vi "02_CheckoutBook.vi"() -> ()   [LabVIEW 2020]
uses:
  librarian_class/librarian.lvclass
  client_class/client.lvclass
panel:
  out "Recieved Match?":bool
  in  "book title":string="ProjectGutenberg-64317-TheGreatGatsby.txt"
  out "book contents":string
  in  "timeout in ms (-1)":i32=-1
  out "client error out":errorcluster
  out "lib error out":errorcluster
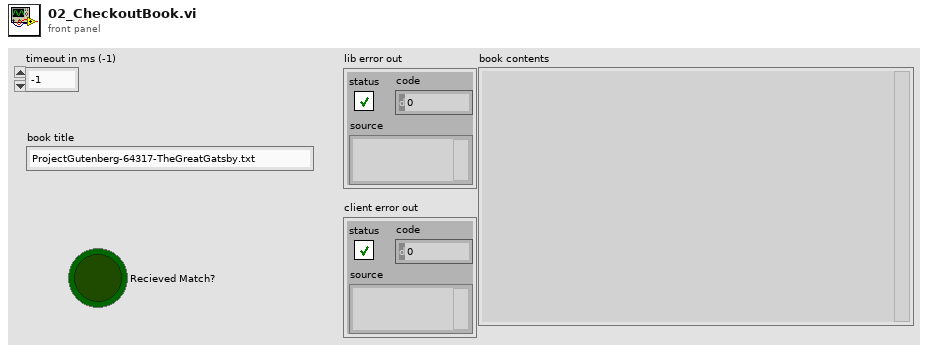
[diagram p1: front panel]
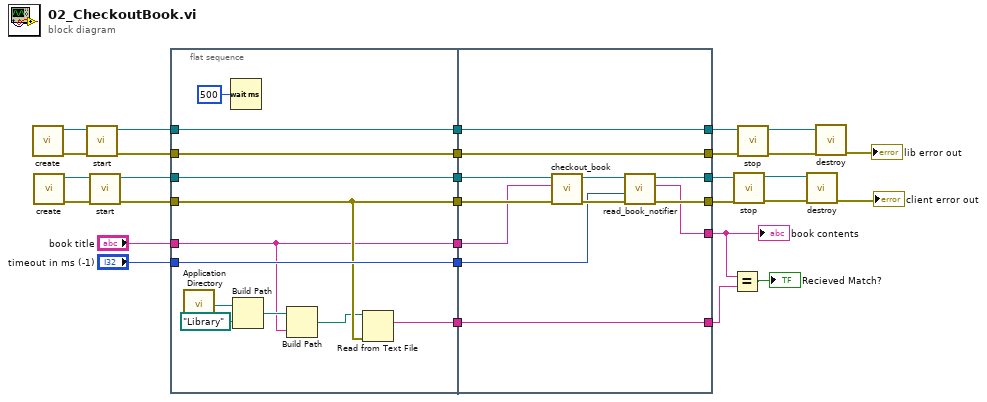
[diagram p0: block diagram]
diagram:
  n1 = call "create.vi"() -> ("error out"=w29:errorcluster, "librarian_sm out"=w30:refnum<class "librarian.lvclass">)  [unwired: 10 in]
  n2 = call "create.vi"() -> ("error out"=w24:errorcluster, "librarian_sm out"=w25:refnum<class "client.lvclass">)  [unwired: 10 in]
  n3 = call "start.vi"("error in (no error)"=w29, "librarian_sm in"=w30) -> ("error out"=w18:errorcluster, "librarian_sm out"=w16:refnum<class "librarian.lvclass">)  [unwired: 8 in]
  n4 = call "start.vi"("error in (no error)"=w24, "librarian_sm in"=w25) -> ("error out"=w20:errorcluster, "librarian_sm out"=w19:refnum<class "client.lvclass">)  [unwired: 8 in]
  n5 = flat-sequence {
    tunnel: "book title" -> [w32]
    tunnel: "timeout in ms (-1)" -> [w39]
    tunnel: w16 -> [w40]
    tunnel: w18 -> [w41]
    tunnel: w19 -> [w42]
    tunnel: w20 -> [w36]
    tunnel: [w36] -> w10
    tunnel: [w42] -> w9
    tunnel: [w41] -> w8
    tunnel: [w40] -> w7
    tunnel: [w39] -> w6
    tunnel: [w32] -> w5
    tunnel: [w35] -> w4
    tunnel: [w52] -> w17
    tunnel: [w51] -> w15
    tunnel: [w49] -> w14
    tunnel: [w47] -> w13
    tunnel: [w45] -> w3
    tunnel: w10 -> [w54]
    tunnel: w9 -> [w53]
    tunnel: w8 -> [w52]
    tunnel: w7 -> [w51]
    tunnel: w6 -> [w46]
    tunnel: w5 -> [w44]
    tunnel: w4 -> [w43]
    tunnel: [w43] -> w2
    frame #0 {
      n6 = call <vilib>:"Application Directory.vi"() -> ("Application Directory"=w37:path)
      n7 = Wait (ms)(milliseconds to wait=u32 500) -> ()  [unwired: 1 out]
      n8 = Build Path(base path=w37, name or relative path=path "Library") -> (appended path=w33:path)
      n9 = Build Path(base path=w33, name or relative path=w32) -> (appended path=w31:path)
      n10 = Read from Text File(file (use dialog)=w31, error in=w36) -> (text=w35:string)  [unwired: 2 in, 3 out]
    }
    frame #1 {
      n11 = call "checkout_book.vi"("error in (no error)"=w54, "book title"=w44, "client in"=w53) -> ("error out"=w48:errorcluster, "client out"=w50:refnum<class "client.lvclass">)  [unwired: 7 in]
      n12 = call "read_book_notifier.vi"("error in (no error)"=w48, "timeout in ms (-1)"=w46, "client in"=w50) -> ("error out"=w47:errorcluster, "book contents"=w45:string, "client out"=w49:refnum<class "client.lvclass">)  [unwired: 6 in]
    }
  }
  n13 = Equal?(x=w3, y=w2) -> (x = y?=→"Recieved Match?":bool)
  n14 = call "stop.vi"("error in (no error)"=w13, "librarian_sm in"=w14) -> ("error out"=w22:errorcluster, "librarian_sm out"=w23:refnum<class "client.lvclass">)  [unwired: 8 in]
  n15 = call "stop.vi"("error in (no error)"=w17, "librarian_sm in"=w15) -> ("error out"=w27:errorcluster, "librarian_sm out"=w28:refnum<class "librarian.lvclass">)  [unwired: 8 in]
  n16 = call "destroy.vi"("error in (no error)"=w22, "librarian_sm in"=w23) -> ("error out"=→"client error out":errorcluster)  [unwired: 8 in, 1 out]
  n17 = call "destroy.vi"("error in (no error)"=w27, "librarian_sm in"=w28) -> ("error out"=→"lib error out":errorcluster)  [unwired: 8 in, 1 out]
  "book contents" <- w3
